vi "beep_pc_speaker_lv821.vi"   [LabVIEW 2018]
doc: "Causes the system to issue an audible tone."
uses:
  Windows/System32/kernel32.dll
panel:
  # "See block diagram for instructions."
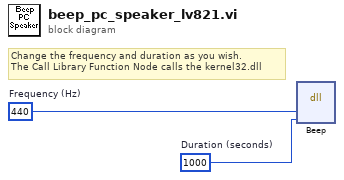
[diagram p0: block diagram]
diagram:
  w1 = 440  # Frequency (Hz)
  w2 = 1000  # Duration (seconds)
  # "Change the frequency and duration as you wish.\nThe Call Library Function Node calls the kernel32.dll"
  n1 = dll-call lib="C:/Windows/System32/KERNEL32.DLL" fn="Beep"(w1, w2) -> ()  [unwired: 6 in, 2 out]
